vi "Reshape volume imaging data-retd.vi"(0 "tdms file ref":refnum<k34>, 1 "TDMS file path & name":path=path "C:/Users/Theo/Desktop/Datasets/140401_17_44_08-rig 3 debugging/Functional imaging TDMS data files/001.tdms", 5 "All header parameters":T1={"Imaging Protocol"=enum."AOL Z-Stack", "Number of POI"=0, "Number of Miniscans"=0, "Number of Trials"=0, "Number of Cycles "=0, "# Averaged Frames"=0, "Laser power (%)"=0, "Pockels"=0.0, "Acquisition Length (sec)"=0.0, "Fill time (us)"=0.0, "POI Dwell time (us)"=0.0, "Miniscan Dwell time per pixel (us)"=0.0, "PMT 1"=0.0, "PMT 2"=0.0, "Back Apperture"=0.0, "Zoom"=0.0, "Frame Size"=200, "Center Frequency"=0.0, "Field of View"=0.0, "DwellTime (us)"=0.0, "Wavelength (nm)"=0.0, "AOL Z"=0.0, "AOL Mode"=enum."Raster", "GridXY"=0.0, "GridZ"=0.0, "TriggerDelay (sec)"=0.0, "Number of Pixels in Miniscan"=0, "Experiment folder path"=path "", "X centre"=0.0, "Y centre"=0.0, "Angle (degrees)"=0.0, "Plane Mode"=0, "Software version"=0.0, "Objective"="Olympus  20X", "MotorZ Calibration"=0, "Pockels Calibration"=0, "Threshold"=[], "Video length (sec)"=0.0, "Frame rate (fps)"=0, "Rectangle ROI length (pixels)"=0, "Rectangle ROI height (pixels)"=0} {"Pockels" format="%#.6g"; "Software version" format="%#.6g"; "Plane Mode" items=["XY Plane", "XZ Plane", "YZ Plane", "arbitraryplane"]; "Angle (degrees)" format="%#.6g"; "Frame Size" items=["100X100"=100, "128X128"=128, "200X200"=200, "256X256"=256, "512X512"=512, "1024x1024"=1024, "2048x2048"=2048]; "Back Apperture" format="%#.6g"; "PMT 2" format="%#.6g"; "PMT 1" format="%#.6g"; "Miniscan Dwell time per pixel (us)" format="%#.6g"; "Zoom" format="%#.6g"; "POI Dwell time (us)" format="%#.6g"; "Acquisition Length (sec)" format="%#.6g"; "Fill time (us)" format="%#.6g"}, 11 "error in (no error)":errorcluster, 12 "Channel to process":enum16{"Red", "Green", "Both"}(ring)) -> (4 "tdms file out":refnum<k34>, 6 "Single channel data":u16[](array[numeric]), 8 "Channel 4D data":u16[][][][](array[numeric]), 10 "Volumetric parameters":T7, 14 "Angles (deg)":dbl[](array[numeric]), 15 "error out":errorcluster)   [LabVIEW 2020]
uses:
  User Interface/Visualisation/Functional Imaging Viewer/SubVIs/Experiment header interface/Typedefs/Header parameters cluster-ALL-retd.ctl
  Typedefs/Imaging Protocols enum.ctl
  Typedefs/Frame Size.ctl
  Typedefs/AOL modes.ctl
  Typedefs/Plane Mode.ctl
  Typedefs/Objective selector control enum.ctl
panel:
  in  "Channel to process":enum16{"Red", "Green"}(ring)
  out "Points in each volume or trial (fractional)":dbl
  out "Points Mismatch":bool
  out "Resulting number of points":i32
  out "Points in each volume or trial":i32
  out "Points in all volumes":i32
  out "Channel size(s)":i32[](array[numeric])
  # "<---This should be an integer. If it is not review the logic inside this VI is suitable"
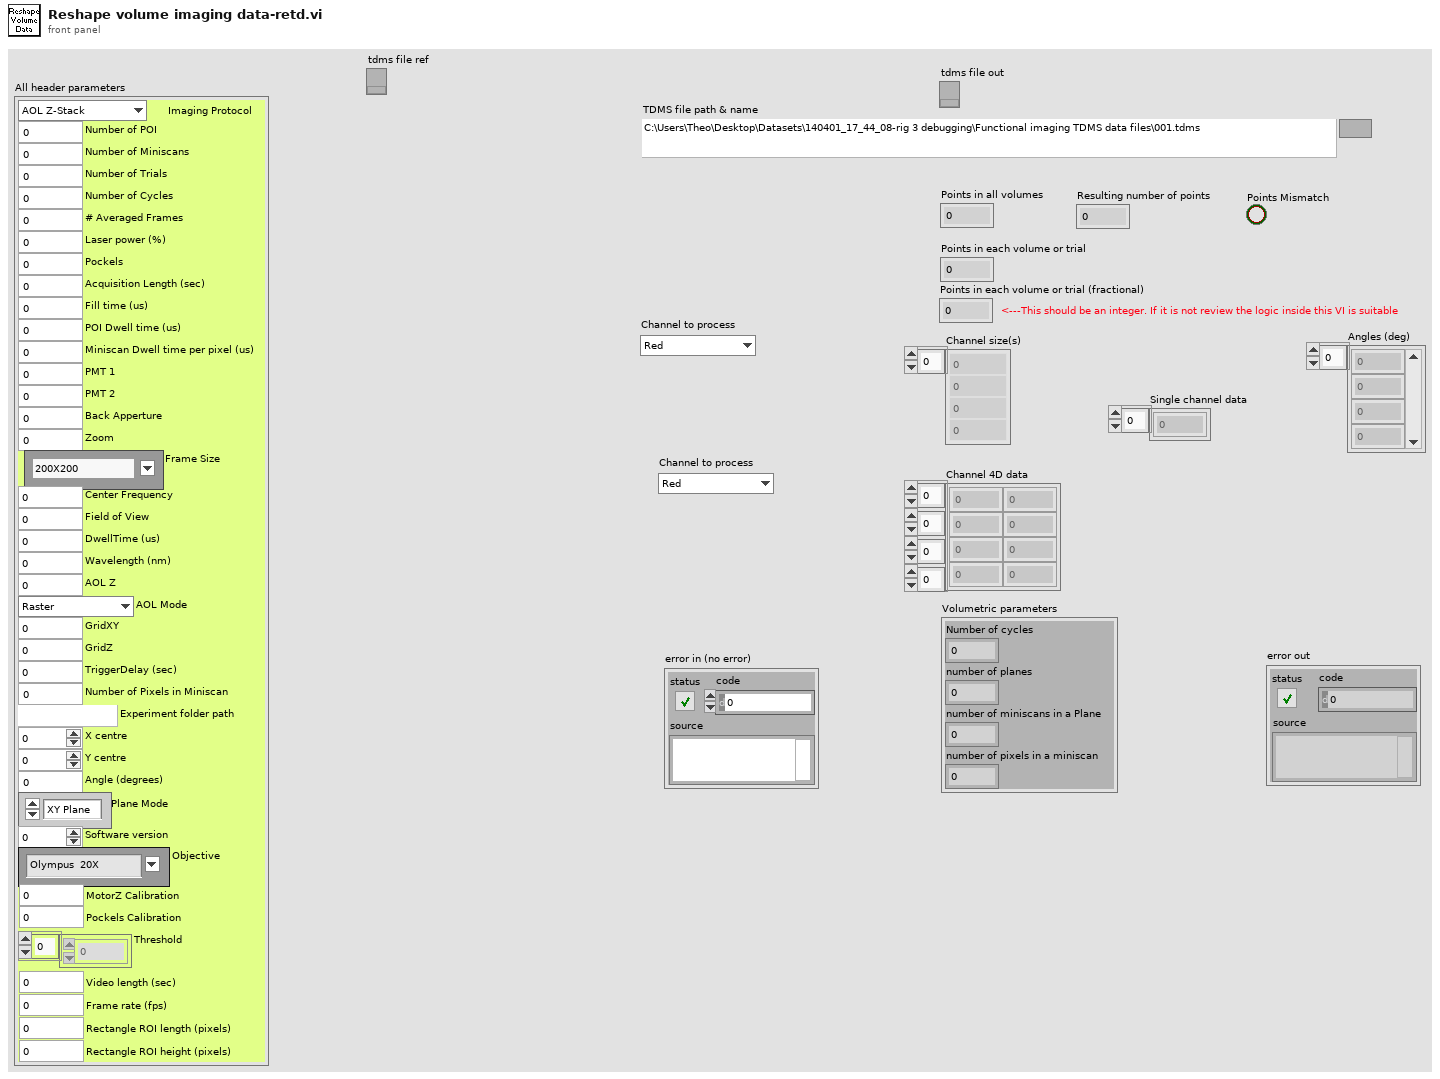
[diagram p1: front panel]
types:
  T1 = typedef "Header parameters cluster-ALL-retd.ctl" = cluster{"Imaging Protocol":T2, "Number of POI":u16, "Number of Miniscans":u16, "Number of Trials":u16, "Number of Cycles ":u64, "# Averaged Frames":u16, "Laser power (%)":u8, "Pockels":dbl, "Acquisition Length (sec)":dbl, "Fill time (us)":dbl, "POI Dwell time (us)":dbl, "Miniscan Dwell time per pixel (us)":dbl, "PMT 1":dbl, "PMT 2":dbl, "Back Apperture":dbl, "Zoom":dbl, "Frame Size":T3, "Center Frequency":dbl, "Field of View":dbl, "DwellTime (us)":dbl, "Wavelength (nm)":dbl, "AOL Z":dbl, "AOL Mode":T4, "GridXY":dbl, "GridZ":dbl, "TriggerDelay (sec)":dbl, "Number of Pixels in Miniscan":u16, "Experiment folder path":path, "X centre":dbl, "Y centre":dbl, "Angle (degrees)":dbl, "Plane Mode":T5, "Software version":dbl, "Objective":T6, "MotorZ Calibration":u32, "Pockels Calibration":u32, "Threshold":u16[], "Video length (sec)":dbl, "Frame rate (fps)":u8, "Rectangle ROI length (pixels)":u16, "Rectangle ROI height (pixels)":u16}
  T2 = typedef "Imaging Protocols enum.ctl" = enum16{"AOL Z-Stack", "Motor Z Stack", "Functional Acquisition", "Single Plane Acquisition", "Volume Acquisition", "Live Imaging", "Live Plane Imaging", "Live Volume Imaging"}
  T3 = typedef "Frame Size.ctl" = u16
  T4 = typedef "AOL modes.ctl" = enum16{"Raster", "Structural", "Pointing", "Mini Scan", "Alignment"}
  T5 = typedef "Plane Mode.ctl" = u16
  T6 = typedef "Objective selector control enum.ctl" = string
  T7 = cluster{"Number of cycles":i32, "number of planes":i32, "number of miniscans in a Plane":i32, "number of pixels in a miniscan":i32}
  T8 = cluster{"Number of trials/volumes":i32, "number of planes":i32, "number of miniscans in a Plane":i32, "number of pixels in a miniscan":i32}
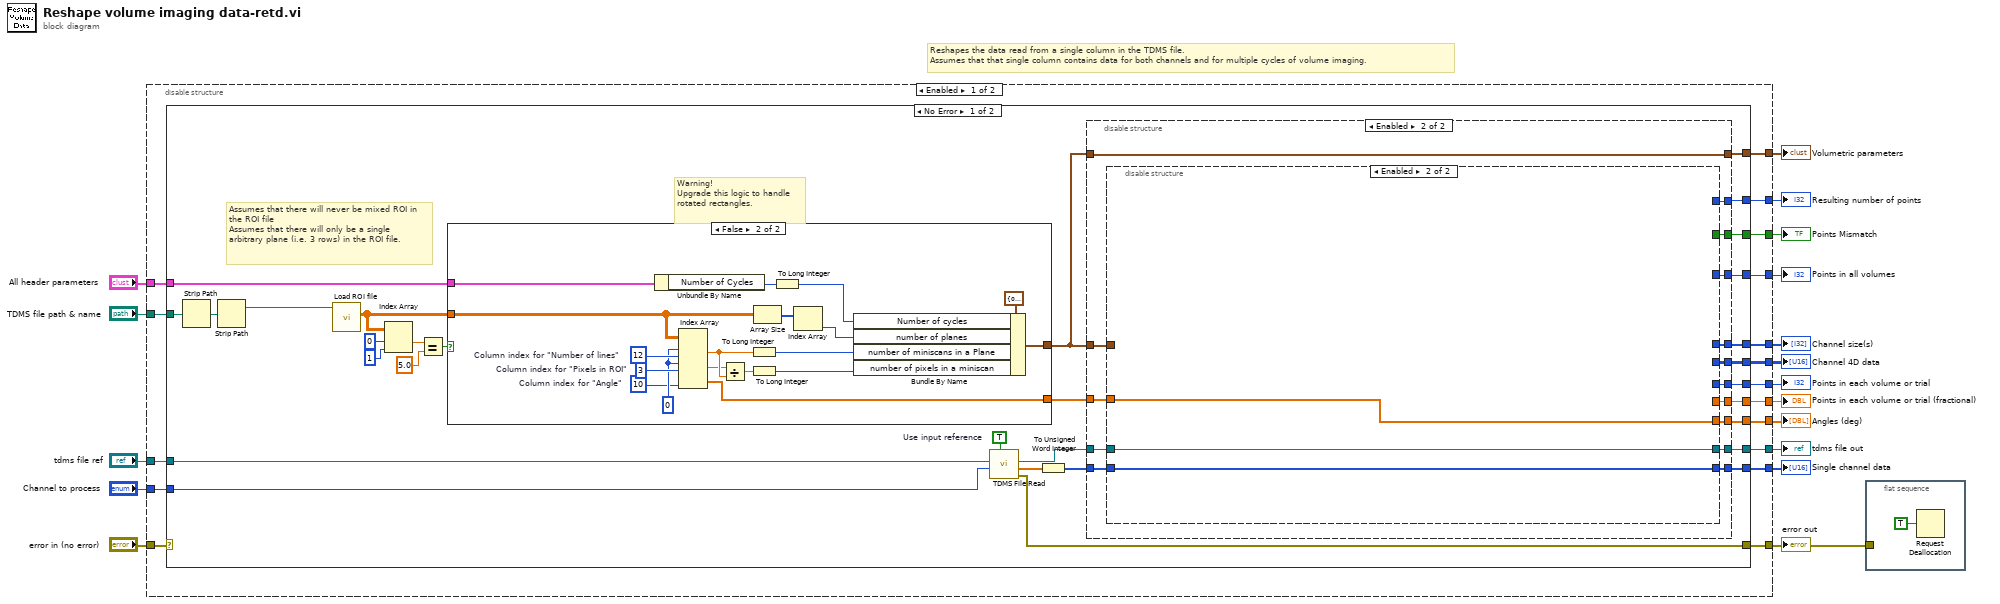
[diagram p0: block diagram]
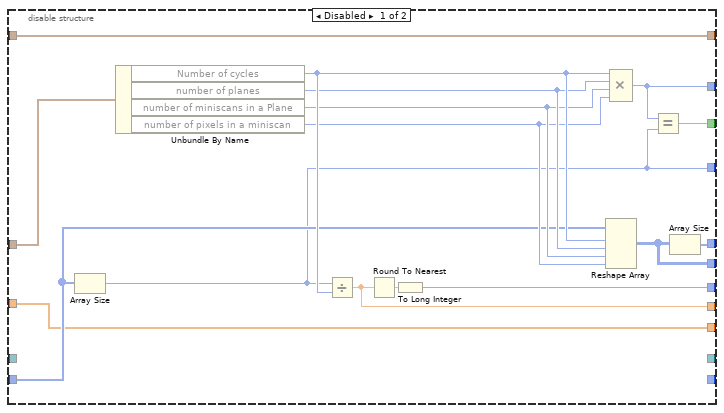
[diagram p2: hidden frame]
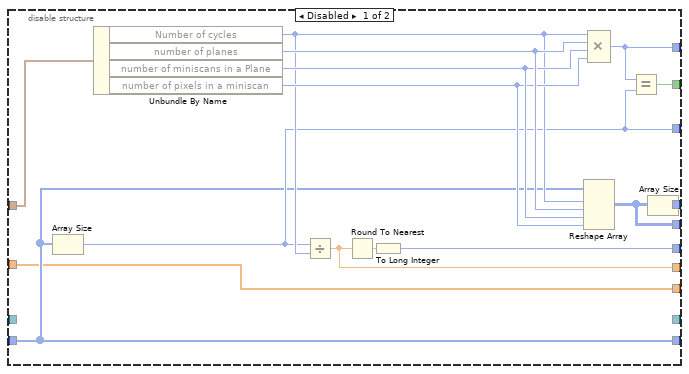
[diagram p3: hidden frame]
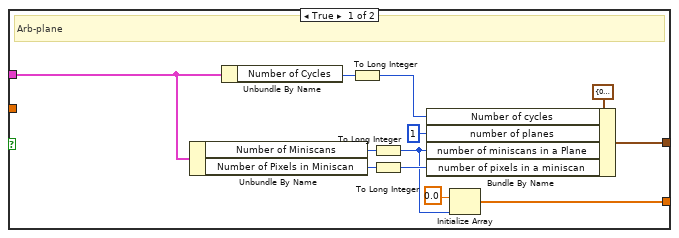
[diagram p4: hidden frame]
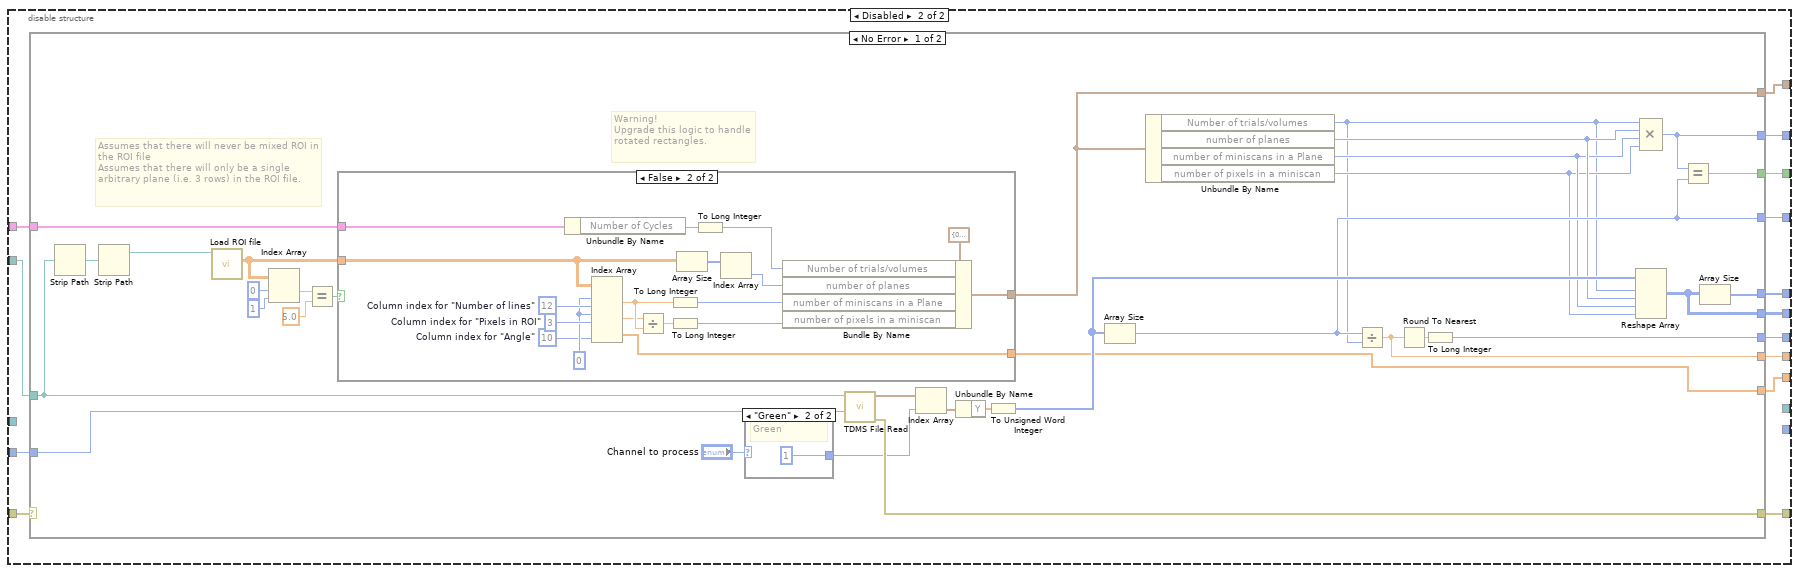
[diagram p6: hidden frame]
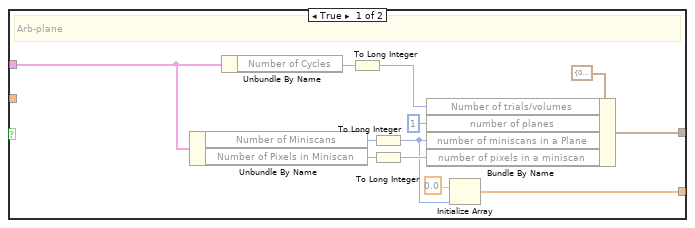
[diagram p7: hidden frame]
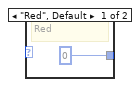
[diagram p8: hidden frame]
diagram:
  # "Reshapes the data read from a single column in the TDMS file.\nAssumes that that single column contains data for both channels and for multiple cycles of volume imaging."
  n1 = disable-structure shown="Enabled" {
    disable-tunnel: [w34 w158] -> w17
    disable-tunnel: "TDMS file path & name" -> [w33 w157]
    disable-tunnel: [w32 w156] -> w15
    disable-tunnel: [w31 w155] -> w14
    disable-tunnel: [w30 w154] -> w13
    disable-tunnel: "error in (no error)" -> [w29 w153]
    disable-tunnel: [w28 w152] -> w11
    disable-tunnel: [w27 w151] -> w10
    disable-tunnel: [w26 w150] -> w9
    disable-tunnel: "All header parameters" -> [w25 w149]
    disable-tunnel: [w24 w148] -> w7
    disable-tunnel: [w23 w147] -> w6
    disable-tunnel: [w22 w146] -> w5
    disable-tunnel: "Channel to process" -> [w21 w145]
    disable-tunnel: [w20 _] -> w3
    disable-tunnel: "tdms file ref" -> [w19 _]
    disable-tunnel: [w18 _] -> w1
    frame Enabled {
      n2 = case shown="No Error" w29 {
        selector: w29 -> [_ w144]
        tunnel: [w64 _] -> w34
        tunnel: w33 -> [w58 _]
        tunnel: [w63 _] -> w32
        tunnel: [w62 _] -> w31
        tunnel: [w61 _] -> w30
        tunnel: [w57 w144] -> w28
        tunnel: w25 -> [w50 _]
        tunnel: [w40 _] -> w26
        tunnel: [w44 _] -> w27
        tunnel: [w48 _] -> w24
        tunnel: [w47 _] -> w23
        tunnel: [w46 _] -> w22
        tunnel: w21 -> [w43 _]
        tunnel: [w42 _] -> w20
        tunnel: w19 -> [w38 _]
        tunnel: [w35 _] -> w18
        frame No Error {
          w39 = TRUE  # Use input reference
          # "Assumes that there will never be mixed ROI in the ROI file\nAssumes that there will only be a single arbitrary plane (i.e. 3 rows) in the ROI file."
          # "Warning!\nUpgrade this logic to handle rotated rectangles."
          n3 = Strip Path(path=w58) -> (stripped path=w59:path)  [unwired: 1 out]
          n4 = Strip Path(path=w59) -> (stripped path=w60:path)  [unwired: 1 out]
          n5 = call "Load ROI file.vi"("Experiment data folder path"=w60) -> ("ROI Data (header removed)"=w56:dbl[][])  [unwired: 7 in, 3 out]
          n6 = Index Array(array=w56, index (row)=0, index (col)=1 ("disabled index (col)")) -> (element=w53:dbl)
          n7 = Equal?(x=w53, y=5.0) -> (x = y?=w51:bool)
          n8 = case shown="False" w51 {
            tunnel: [w125 w139] -> w41
            tunnel: [w121 w130] -> w45
            tunnel: w56 -> [_ w131]
            tunnel: w50 -> [w117 w127]
            frame True {
              # "Arb-plane"
              n9 = Unbundle By Name(w117) -> ("Number of Miniscans"=w116:u16, "Number of Pixels in Miniscan"=w115:u16)
              n10 = Unbundle By Name(w117) -> ("Number of Cycles"=w119:u64)
              n11 = To Long Integer(number=w119) -> (32bit integer=w118:i32)
              n12 = To Long Integer(number=w116) -> (32bit integer=w120:i32)
              n13 = To Long Integer(number=w115) -> (32bit integer=w123:i32)
              n14 = Bundle By Name(cluster=T7 {"Number of cycles"=0, "number of planes"=0, "number of miniscans in a Plane"=0, "number of pixels in a miniscan"=0} ("Parameters Cluster"), "Number of cycles"=w118, "number of planes"=1, "number of miniscans in a Plane"=w120, "number of pixels in a miniscan"=w123) -> (w125:T7)
              n15 = Initialize Array(0.0 ("element"), w120) -> (w121:dbl[])
            }
            frame False {
              w136 = 10  # Column index for "Angle"
              w137 = 0 ("disabled index (row)")
              w142 = 3  # Column index for "Pixels in ROI"
              w143 = 12  # Column index for "Number of lines"
              n16 = Unbundle By Name(w127) -> ("Number of Cycles"=w129:u64)
              n17 = Index Array(array=w131, index (row) #1=w137, index (col) #1=w143, index (row) #2=w137, index (col) #2=w142, index (col) #3=w136) -> (element #1=w135:dbl, element #2=w134:dbl, element #3=w130:dbl[])  [unwired: 1 in]
              n18 = Divide(x=w134, y=w135) -> (x/y=w138:dbl)
              n19 = To Long Integer(number=w135) -> (32bit integer=w133:i32)
              n20 = To Long Integer(number=w138) -> (32bit integer=w132:i32)
              n21 = Array Size(array=w131) -> (size(s)=w141:i32[])
              n22 = To Long Integer(number=w129) -> (32bit integer=w128:i32)
              n23 = Index Array(array=w141) -> (element=w140:i32)  [unwired: 1 in]
              n24 = Bundle By Name(cluster=T7 {"Number of cycles"=0, "number of planes"=0, "number of miniscans in a Plane"=0, "number of pixels in a miniscan"=0} ("Parameters Cluster"), "Number of cycles"=w128, "number of planes"=w140, "number of miniscans in a Plane"=w133, "number of pixels in a miniscan"=w132) -> (w139:T7)
            }
          }
          n25 = call "TDMS File Read.vi"("Use input reference (F)"=w39, "Channel to load"=w43, "tdms file ref"=w38) -> ("Error Out"=w57:errorcluster, "Single channel data"=w37:dbl[], "tdms file out"=w36:refnum<k34>)  [unwired: 4 in, 2 out]
          n26 = To Unsigned Word Integer(number=w37) -> (unsigned 16bit integer=w49:u16[])
          n27 = disable-structure shown="Enabled" {
            disable-tunnel: [w80 w95] -> w64
            disable-tunnel: [w78 w94] -> w63
            disable-tunnel: [w77 w93] -> w62
            disable-tunnel: [w76 w92] -> w61
            disable-tunnel: w41 -> [w65 w88]
            disable-tunnel: w49 -> [w71 w87]
            disable-tunnel: [w70 w91] -> w48
            disable-tunnel: [w69 w90] -> w47
            disable-tunnel: [w68 w89] -> w46
            disable-tunnel: w45 -> [w67 w85]
            disable-tunnel: [w67 w84] -> w44
            disable-tunnel: [_ w86] -> w42
            disable-tunnel: w41 -> [w66 w83]
            disable-tunnel: [w66 w83] -> w40
            disable-tunnel: w36 -> [_ w82]
            disable-tunnel: [_ w81] -> w35
            frame Disabled {
              n28 = Array Size(array=w71) -> (size(s)=w68:i32)
              n29 = Unbundle By Name(w65) -> ("Number of cycles"=w75:i32, "number of planes"=w74:i32, "number of miniscans in a Plane"=w73:i32, "number of pixels in a miniscan"=w72:i32)
              n30 = Divide(x=w68, y=w75) -> (x/y=w69:dbl)
              n31 = Round To Nearest(number=w69) -> (nearest integer value=w79:dbl)
              n32 = To Long Integer(number=w79) -> (32bit integer=w70:i32)
              n33 = Reshape Array(w71, w75, w74, w73, w72) -> (w76:u16[][][][])
              n34 = Compound Arithmetic op=MULTIPLY(w75, w74, w73, w72) -> (w78:i32)
              n35 = Equal?(x=w78, y=w68) -> (x = y?=w77:bool)
              n36 = Array Size(array=w76) -> (size(s)=w80:i32[])
            }
            frame Enabled {
              n37 = disable-structure shown="Enabled" {
                disable-tunnel: [w110 _] -> w95
                disable-tunnel: [w108 _] -> w94
                disable-tunnel: [w107 _] -> w93
                disable-tunnel: [w106 _] -> w92
                disable-tunnel: [w102 _] -> w91
                disable-tunnel: [w101 _] -> w90
                disable-tunnel: [w99 _] -> w89
                disable-tunnel: w88 -> [w98 _]
                disable-tunnel: w87 -> [w97 w113]
                disable-tunnel: [w97 w113] -> w86
                disable-tunnel: w85 -> [w96 w112]
                disable-tunnel: [w96 w112] -> w84
                disable-tunnel: w82 -> [_ w111]
                disable-tunnel: [_ w111] -> w81
                frame Disabled {
                  n38 = Array Size(array=w97) -> (size(s)=w99:i32)
                  n39 = Unbundle By Name(w98) -> ("Number of cycles"=w100:i32, "number of planes"=w105:i32, "number of miniscans in a Plane"=w104:i32, "number of pixels in a miniscan"=w103:i32)
                  n40 = Divide(x=w99, y=w100) -> (x/y=w101:dbl)
                  n41 = Round To Nearest(number=w101) -> (nearest integer value=w109:dbl)
                  n42 = To Long Integer(number=w109) -> (32bit integer=w102:i32)
                  n43 = Reshape Array(w97, w100, w105, w104, w103) -> (w106:u16[][][][])
                  n44 = Compound Arithmetic op=MULTIPLY(w100, w105, w104, w103) -> (w108:i32)
                  n45 = Equal?(x=w108, y=w99) -> (x = y?=w107:bool)
                  n46 = Array Size(array=w106) -> (size(s)=w110:i32[])
                }
                frame Enabled {
                }
              }
            }
          }
        }
        frame Error {
        }
      }
    }
    frame Disabled {
      n47 = case shown="No Error" w153 {
        selector: w153 -> [_ w223]
        tunnel: [w190 _] -> w158
        tunnel: w157 -> [w181 _]
        tunnel: [w186 _] -> w156
        tunnel: [w185 _] -> w155
        tunnel: [w184 _] -> w154
        tunnel: [w179 w223] -> w152
        tunnel: w149 -> [w171 _]
        tunnel: [w180 _] -> w150
        tunnel: [w166 _] -> w151
        tunnel: [w169 _] -> w148
        tunnel: [w168 _] -> w147
        tunnel: [w167 _] -> w146
        tunnel: w145 -> [w159 _]
        frame No Error {
          # "Assumes that there will never be mixed ROI in the ROI file\nAssumes that there will only be a single arbitrary plane (i.e. 3 rows) in the ROI file."
          # "Warning!\nUpgrade this logic to handle rotated rectangles."
          n48 = Strip Path(path=w181) -> (stripped path=w182:path)  [unwired: 1 out]
          n49 = Strip Path(path=w182) -> (stripped path=w183:path)  [unwired: 1 out]
          n50 = call "Load ROI file.vi"("Experiment data folder path"=w183) -> ("ROI Data (header removed)"=w177:dbl[][])  [unwired: 7 in, 3 out]
          n51 = Index Array(array=w177, index (row)=0, index (col)=1 ("disabled index (col)")) -> (element=w174:dbl)
          n52 = Equal?(x=w174, y=5.0) -> (x = y?=w172:bool)
          n53 = case shown="False" w172 {
            tunnel: [w201 w215] -> w180
            tunnel: [w197 w206] -> w166
            tunnel: w177 -> [_ w207]
            tunnel: w171 -> [w193 w203]
            frame True {
              # "Arb-plane"
              n54 = Unbundle By Name(w193) -> ("Number of Miniscans"=w192:u16, "Number of Pixels in Miniscan"=w191:u16)
              n55 = Unbundle By Name(w193) -> ("Number of Cycles"=w195:u64)
              n56 = To Long Integer(number=w195) -> (32bit integer=w194:i32)
              n57 = To Long Integer(number=w192) -> (32bit integer=w196:i32)
              n58 = To Long Integer(number=w191) -> (32bit integer=w199:i32)
              n59 = Bundle By Name(cluster=T8 {"Number of trials/volumes"=0, "number of planes"=0, "number of miniscans in a Plane"=0, "number of pixels in a miniscan"=0} ("Parameters Cluster"), "Number of trials/volumes"=w194, "number of planes"=1, "number of miniscans in a Plane"=w196, "number of pixels in a miniscan"=w199) -> (w201:T8)
              n60 = Initialize Array(0.0 ("element"), w196) -> (w197:dbl[])
            }
            frame False {
              w212 = 10  # Column index for "Angle"
              w213 = 0 ("disabled index (row)")
              w219 = 3  # Column index for "Pixels in ROI"
              w220 = 12  # Column index for "Number of lines"
              n61 = Unbundle By Name(w203) -> ("Number of Cycles"=w205:u64)
              n62 = Index Array(array=w207, index (row) #1=w213, index (col) #1=w220, index (row) #2=w213, index (col) #2=w219, index (col) #3=w212) -> (element #1=w211:dbl, element #2=w210:dbl, element #3=w206:dbl[])  [unwired: 1 in]
              n63 = Divide(x=w210, y=w211) -> (x/y=w214:dbl)
              n64 = To Long Integer(number=w211) -> (32bit integer=w209:i32)
              n65 = To Long Integer(number=w214) -> (32bit integer=w208:i32)
              n66 = Array Size(array=w207) -> (size(s)=w218:i32[])
              n67 = To Long Integer(number=w205) -> (32bit integer=w204:i32)
              n68 = Index Array(array=w218) -> (element=w217:i32)  [unwired: 1 in]
              n69 = Bundle By Name(cluster=T8 {"Number of trials/volumes"=0, "number of planes"=0, "number of miniscans in a Plane"=0, "number of pixels in a miniscan"=0} ("Parameters Cluster"), "Number of trials/volumes"=w204, "number of planes"=w217, "number of miniscans in a Plane"=w209, "number of pixels in a miniscan"=w208) -> (w215:T8)
            }
          }
          n70 = case shown="\"Green\"" "Channel to process" {
            tunnel: [0 ("index") 1 ("index")] -> w178
            frame "Red", Default {
              # "Red"
            }
            frame "Green" {
              # "Green"
            }
          }
          n71 = call "TDMS File Read.vi"("Channel to load"=w159, "File Path"=w181) -> ("Error Out"=w179:errorcluster, "Data"=w189:waveform(dbl)[])  [unwired: 5 in, 3 out]
          n72 = Index Array(array=w189, index=w178) -> (element=w188:waveform(dbl))
          n73 = Unbundle By Name ("Get Waveform Components")(w188) -> ("Y"=w187:dbl[])
          n74 = To Unsigned Word Integer(number=w187) -> (unsigned 16bit integer=w170:u16[])
          n75 = Array Size(array=w170) -> (size(s)=w167:i32)
          n76 = Unbundle By Name(w180) -> ("Number of trials/volumes"=w161:i32, "number of planes"=w164:i32, "number of miniscans in a Plane"=w163:i32, "number of pixels in a miniscan"=w162:i32)
          n77 = Divide(x=w167, y=w161) -> (x/y=w168:dbl)
          n78 = Round To Nearest(number=w168) -> (nearest integer value=w165:dbl)
          n79 = To Long Integer(number=w165) -> (32bit integer=w169:i32)
          n80 = Reshape Array(w170, w161, w164, w163, w162) -> (w184:u16[][][][])
          n81 = Compound Arithmetic op=MULTIPLY(w161, w164, w163, w162) -> (w186:i32)
          n82 = Equal?(x=w186, y=w167) -> (x = y?=w185:bool)
          n83 = Array Size(array=w184) -> (size(s)=w190:i32[])
        }
        frame Error {
        }
      }
    }
  }
  "Channel size(s)" <- w17
  "Resulting number of points" <- w15
  "Points Mismatch" <- w14
  "Channel 4D data" <- w13
  "error out" <- w11
  "Volumetric parameters" <- w9
  "Angles (deg)" <- w10
  "Points in each volume or trial" <- w7
  "Points in each volume or trial (fractional)" <- w6
  "Points in all volumes" <- w5
  "Single channel data" <- w3
  "tdms file out" <- w1
  n84 = flat-sequence {
    tunnel: w11 -> [_]
    frame #0 {
      n85 = Request Deallocation(TRUE ("flag")) -> ()
    }
  }
